vi "H5Tenum_nameof.vi"(6 "error in (no error)":errorcluster, 8 "Member Value":variant, 9 "HDF5 Type Ref":T1) -> (0 "error out":errorcluster, 2 "Member Name":string, 3 "HDF5 Type Ref out":T1)   [LabVIEW 2017]
doc: "Returns the symbol name corresponding to a specified member \n of an enumeration datatype."
uses:
  <vilib>/UPVI/lvhdf5/library.llb/HDF5 Ref.ctl
  <vilib>/UPVI/lvhdf5/hdf5.dll
panel:
  # "LVHDF5 Toolkit\nCopyright (c) 2005-2013 by Jason D. Sommerville\nCopyright (c) 2014 by UPVI, LLC.\n\nThis use and distribution of this file is governed by the terms found in \nLICENSE.txt distributed with this toolkit and installed at\n <user.lib>\\_lvhdf5\\LICENSE.txt"
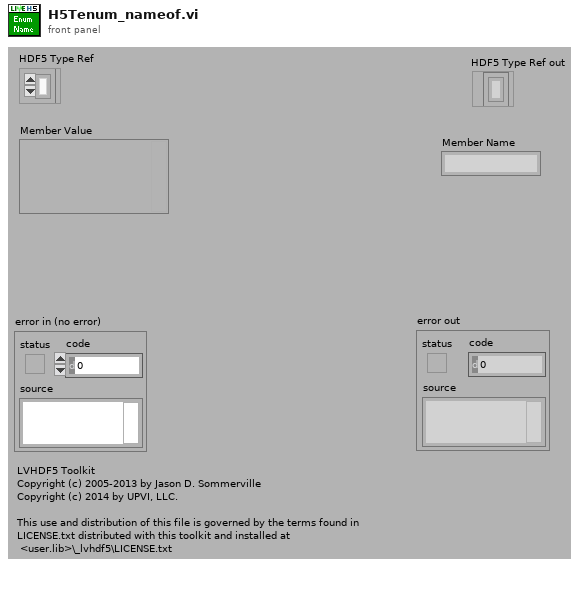
[diagram p1: front panel]
types:
  T1 = typedef "HDF5 Ref.ctl" = refnum<k1>
  T2 = typedef "Type Descriptor Enumeration__ogtk.ctl" = enum8{"<Null>", "I8", "I16", "I32", "I64", "U8", "U16", "U32", "U64", "SGL", "DBL", "EXT", "CSG", "CDB", "CXT", "0x0F", "0x10", "0x11", "0x12", "0x13", "0x14", "Enum U8", "Enum U16", "Enum U32", "Enum U64", "SGL PQ", "DBL PQ", "EXT PQ", "CSG PQ", "CDB PQ", "CXT PQ", "0x1F", "0x20", "Boolean", "0x22", "0x23", "0x24", "0x25", "0x26", "0x27", "0x28", "0x29", "0x2A", "0x2B", "0x2C", "0x2D", "0x2E", "0x2F", "String", "0x31", "Path", "Pict", "0x34", "0x35", "0x36", "DAQ", "0x38", "0x39", "0x3A", "0x3B", "0x3C", "0x3D", "0x3E", "0x3F", "Array", "0x41", "0x42", "0x43", "0x44", "0x45", "0x46", "0x47", "0x48", "0x49", "0x4A", "0x4B", "0x4C", "0x4D", "0x4E", "0x4F", "Cluster", "0x51", "0x52", "Variant", "Waveform", "0x55", "0x56", "0x57", "0x58", "0x59", "0x5A", "0x5B", "0x5C", "0x5D", "0x5E", "0x5F", "0x60", "0x61", "0x62", "0x63", "0x64", "0x65", "0x66", "0x67", "0x68", "0x69", "0x6A", "0x6B", "0x6C", "0x6D", "0x6E", "0x6F", "Refnum"}
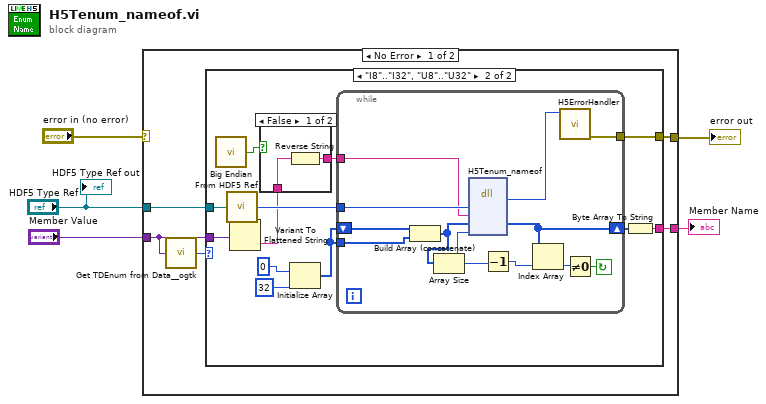
[diagram p0: block diagram]
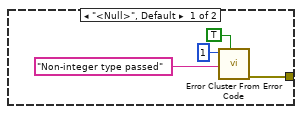
[diagram p2: hidden frame]
diagram:
  n1 = case shown="No Error" "error in (no error)" {
    selector: "error in (no error)" -> [_ w42]
    tunnel: [w10 w42] -> w4
    tunnel: "HDF5 Type Ref" -> [w9 _]
    tunnel: "Member Value" -> [w7 _]
    tunnel: [w6 _] -> w1
    frame No Error {
      n2 = call <userlib>:"Get TDEnum from Data__ogtk.vi"("Data"=w7) -> ("Type Descriptor Enumeration"=w8:T2)  [unwired: 4 in]
      n3 = case shown="\"I8\"..\"I32\", \"U8\"..\"U32\"" w8 {
        tunnel: [w14 w22] -> w10
        tunnel: w9 -> [_ w26]
        tunnel: w7 -> [_ w21]
        tunnel: [_ w23] -> w6
        frame "<Null>", Default {
          n4 = call <vilib>:"Error Cluster From Error Code.vi"("show call chain? (False)"=TRUE, "error message (\"\")"="Non-integer type passed" ("error message (\"\")"), "error code (0)"=1) -> ("error out"=w14:errorcluster)  [unwired: 6 in]
        }
        frame "I8".."I32", "U8".."U32" {
          n5 = call <vilib>:"Big Endian.vi"() -> ("big endian"=w20:bool)
          n6 = call <vilib>:"From HDF5 Ref.vi"("HDF5 Ref"=w26) -> ("I32"=w25:i32)
          n7 = Variant To Flattened String(Variant=w21) -> (data string=w19:string)  [unwired: 1 out]
          n8 = case shown="False" w20 {
            tunnel: w19 -> [w28 w29]
            tunnel: [w27 w29] -> w18
            frame False {
              n9 = Reverse String(1:w28) -> (0:w27:string)
            }
            frame True {
            }
          }
          n10 = Initialize Array(u8 0, 32 ("dimension size")) -> (w15:u8[])
          n11 = while {
            tunnel: w25 -> [w40]
            shift-right: [w39] -> w24
            shift-left: w15 -> [w34]
            tunnel: [w36] -> w22
            tunnel: w18 -> [w35]
            tunnel: w15 -> [w33]
            stop <- w37 continue-if-true
            n12 = Build Array (concatenate)(w34, w33) -> (w32:u8[])
            n13 = Array Size(array=w32) -> (size(s)=w31:i32)
            n14 = dll-call lib="C:/Program Files/National Instruments/LabVIEW 2017/vi.lib/UPVI/lvhdf5/hdf5.dll" fn="H5Tenum_nameof"("type_id"=w40, "value"=w35, "name"=w32, "size"=w31) -> ("return type"=w41:i32, "name"=w39:u8[])  [unwired: 6 in, 2 out]
            n15 = Decrement(x=w31) -> (x-1=w30:i32)
            n16 = Index Array(array=w39, index=w30) -> (element=w38:u8)
            n17 = call <vilib>:"H5ErrorHandler.vi"("herr_t"=w41) -> ("error out"=w36:errorcluster)  [unwired: 4 in, 4 out]
            n18 = Not Equal To 0?(x=w38) -> (x != 0?=w37:bool)
          }
          n19 = Byte Array To String(unsigned byte array=w24) -> (string=w23:string)
        }
      }
    }
    frame Error {
    }
  }
  "error out" <- w4
  "Member Name" <- w1
  "HDF5 Type Ref out" <- "HDF5 Type Ref"
